vi "KB-CalConcentrieity.vi"(0 "Image  In":T5(plugin-control), 1 "ROI Descriptor (Otter-Find Circular Edge)":T1={"Global Rectangle"=[686, 409, 1084, 806], "Contours"=[{"ID"=enum."External", "Type"=7, "Coordinates"=[884, 607, 109, 198, 0, 0]}]} {"Contours"."Type" items=["No Selection", "Point", "Line", "Rectangle", "Oval", "Polygon", "Freehand Region", "Annulus", "Unused2", "Unused3", "Broken Line", "Freehand Line", "Rotated Rectangle"]}, 2 "Options (Otter-Find Circular Edge)":T4={"Search  Direction"=0, "Edge Options"={"Edge Polarity"=0, "Kernel Size"=13, "Width"=13, "Minimum Edge Strength"=53.0, "Interpolation Type"=enum."Bilinear Fixed", "Data Processing Method"=enum."Average"}, "Show Search Area"=TRUE, "Show Search Lines"=TRUE, "Show Edges Found"=TRUE, "Show Result"=TRUE, "Search Area Color"=65280, "Search Lines Color"=255, "Edge Locations Color"=16776960, "Result Color"=16711680, "Overlay Group Name"=""} {"Search  Direction" items=["Outside to Inside", "Inside to Outside"]; "Edge Options"."Edge Polarity" items=["All Edges", "Rising Edges", "Falling Edges"]; "Edge Options"."Minimum Edge Strength" format="%.2f"; "Edge Options"."Width" step=2; "Edge Options"."Kernel Size" step=2}, 3 "ROI Descriptor (Inner Find Circular Edge 2)":T1={"Global Rectangle"=[775, 498, 995, 717], "Contours"=[{"ID"=enum."External", "Type"=7, "Coordinates"=[884, 607, 51, 109, 0, 0]}]} {"Contours"."Type" items=["No Selection", "Point", "Line", "Rectangle", "Oval", "Polygon", "Freehand Region", "Annulus", "Unused2", "Unused3", "Broken Line", "Freehand Line", "Rotated Rectangle"]}, 4 "Options (Inner Find Circular Edge 2)":T4={"Search  Direction"=0, "Edge Options"={"Edge Polarity"=0, "Kernel Size"=13, "Width"=13, "Minimum Edge Strength"=72.0, "Interpolation Type"=enum."Bilinear Fixed", "Data Processing Method"=enum."Average"}, "Show Search Area"=TRUE, "Show Search Lines"=TRUE, "Show Edges Found"=TRUE, "Show Result"=TRUE, "Search Area Color"=65280, "Search Lines Color"=255, "Edge Locations Color"=16776960, "Result Color"=16711680, "Overlay Group Name"=""} {"Search  Direction" items=["Outside to Inside", "Inside to Outside"]; "Edge Options"."Edge Polarity" items=["All Edges", "Rising Edges", "Falling Edges"]; "Edge Options"."Minimum Edge Strength" format="%.2f"; "Edge Options"."Width" step=2; "Edge Options"."Kernel Size" step=2}, 5 "error in":errorcluster, 6 "Row Select":string(combo)="Item1", 7 "Range (Threshold 1)":cluster{"Lower value":sgl, "Upper value":sgl}={"Lower value"=218.0, "Upper value"=255.0}, 8 "相机分辨率":string) -> (13 "U I Center":cluster{"X":sgl, "Y":sgl}[](array[cluster]), 14 "Image  Out":T5(plugin-control), 16 "Concentrieity":string, 17 "color":string, 18 "New Inneer ROI":T1, 19 "error out":errorcluster)   [LabVIEW 2015]
uses:
  <vilib>/vision/Measure.llb/Edge Options.ctl
  <vilib>/vision/Measure.llb/Edge Polarity.ctl
  Global System.vi
panel:
  out "New Inneer ROI 2":T1
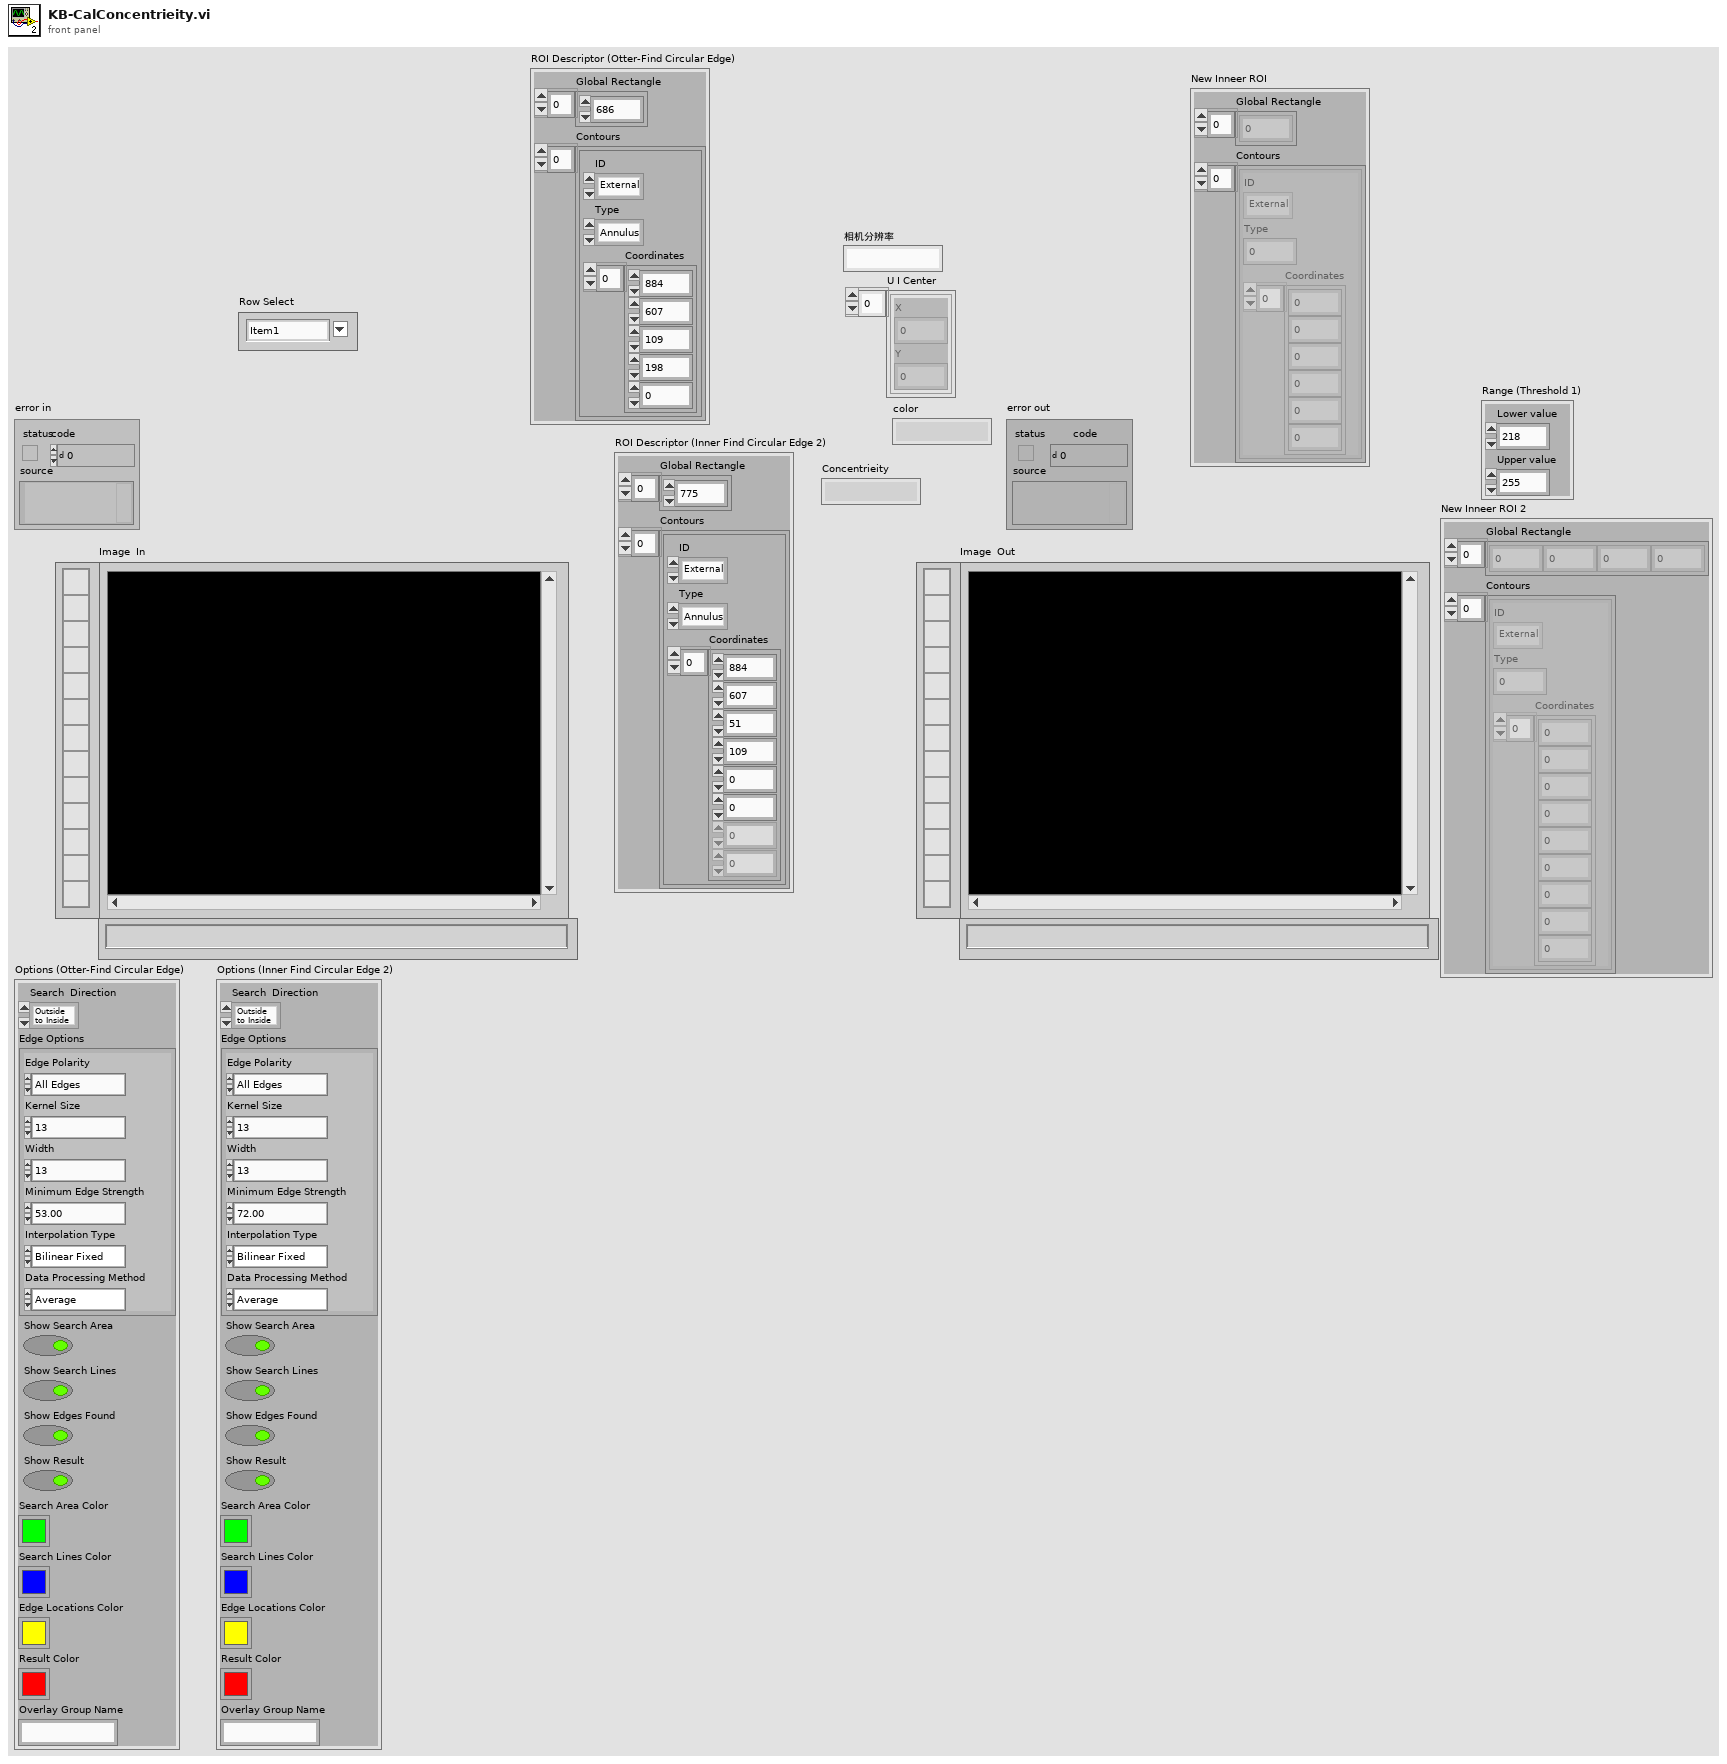
[diagram p1: front panel]
types:
  T1 = cluster{"Global Rectangle":i32[], "Contours":cluster{"ID":enum32{"External", "Internal"}, "Type":u32, "Coordinates":i32[]}[]}
  T2 = typedef "Edge Options.ctl" = cluster{"Edge Polarity":T3, "Kernel Size":u32, "Width":u32, "Minimum Edge Strength":sgl, "Interpolation Type":enum32{"Zero Order", "Bilinear", "Quadratic", "Cubic", "Bilinear Fixed"}, "Data Processing Method":enum32{"Average", "Median"}}
  T3 = typedef "Edge Polarity.ctl" = u32
  T4 = cluster{"Search  Direction":u32, "Edge Options":T2, "Show Search Area":bool, "Show Search Lines":bool, "Show Edges Found":bool, "Show Result":bool, "Search Area Color":u32, "Search Lines Color":u32, "Edge Locations Color":u32, "Result Color":u32, "Overlay Group Name":string}
  T5 = typedef "IMAQ Image.ctl" = refnum<image>
  T6 = cluster{"Left":i32, "Top":i32, "Right":i32, "Bottom":i32}
  T7 = typedef "Image Type" = u32
  T8 = cluster{"ID":enum32{"External", "Internal"}, "Type":u32, "Coordinates":i32[]}
  T9 = cluster{"Process":enum16{"Get First Edge", "Get First + Last Edge", "Get All Edges", "Get Best Edge"}, "Step Size":i32, "Max Pixel Radius":i32}
  T10 = cluster{"Center (Pixels)":cluster{"X":sgl, "Y":sgl}, "Radius (Pixels)":dbl, "Center (Real-World)":cluster{"X":sgl, "Y":sgl}, "Radius (Real-World)":dbl, "Roundness (Real-World)":dbl, "Average Strength":dbl, "Average SNR (dB)":dbl}
  T11 = cluster{"left":dbl, "top":dbl, "right":dbl, "bottom":dbl}
  T12 = cluster{"ID":enum32{"External", "Internal"}, "Type":u32, "Coordinates":i32[]}[]
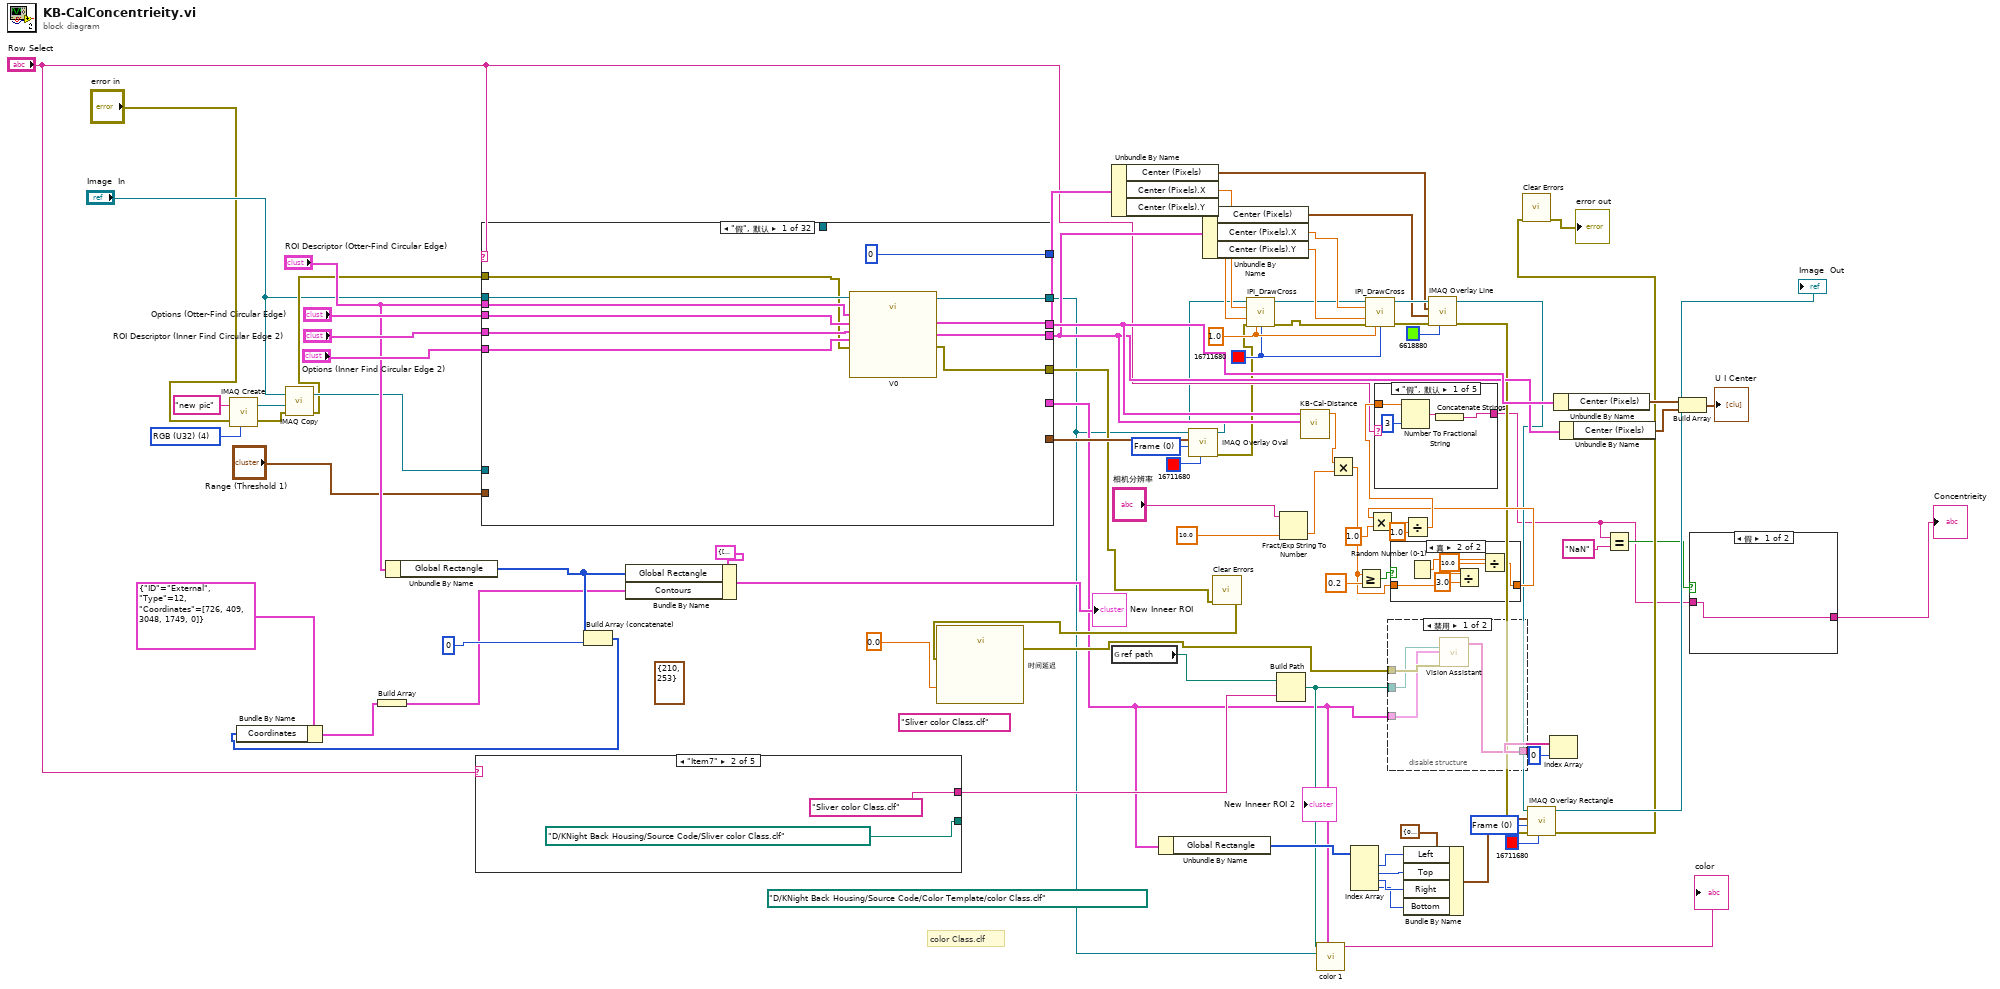
[diagram p0: block diagram]
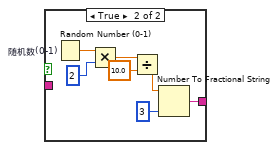
[diagram p2: hidden frame]
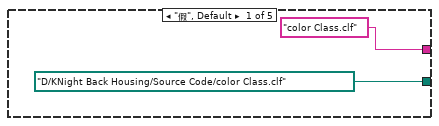
[diagram p4: hidden frame]
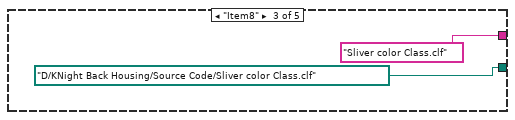
[diagram p5: hidden frame]
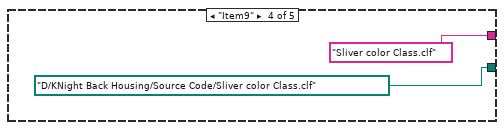
[diagram p6: hidden frame]
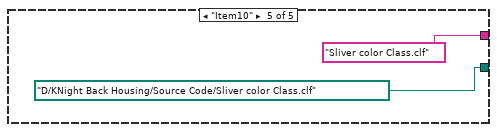
[diagram p7: hidden frame]
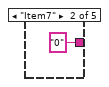
[diagram p9: hidden frame]
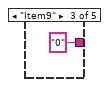
[diagram p10: hidden frame]
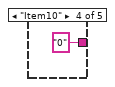
[diagram p11: hidden frame]
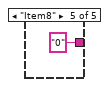
[diagram p12: hidden frame]
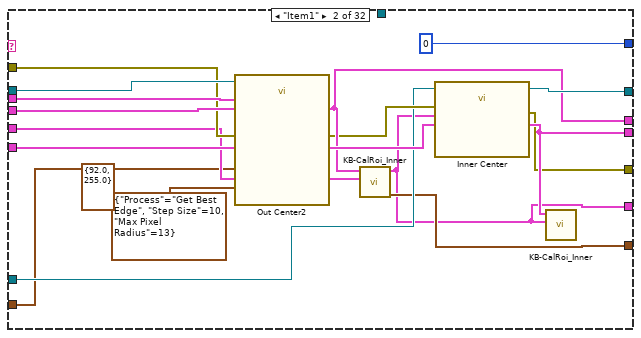
[diagram p13: hidden frame]
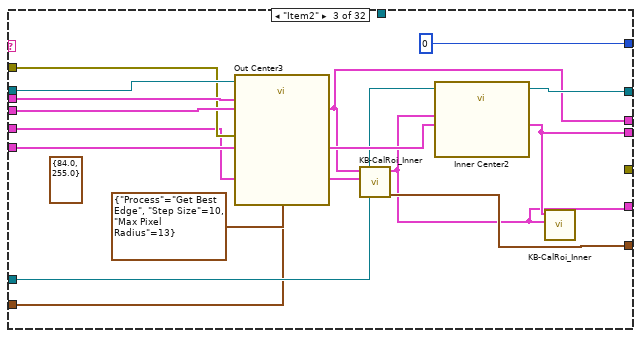
[diagram p14: hidden frame]
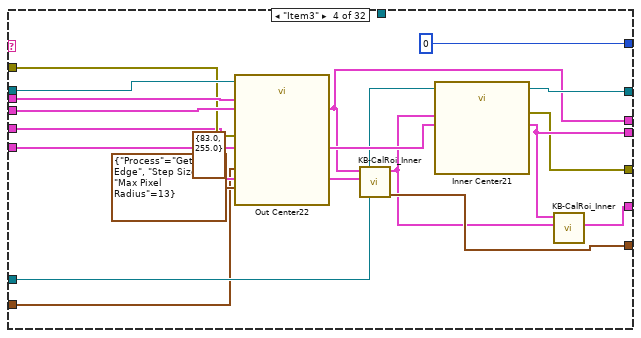
[diagram p15: hidden frame]
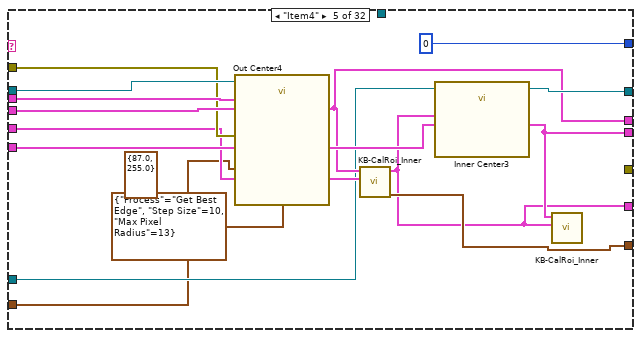
[diagram p16: hidden frame]
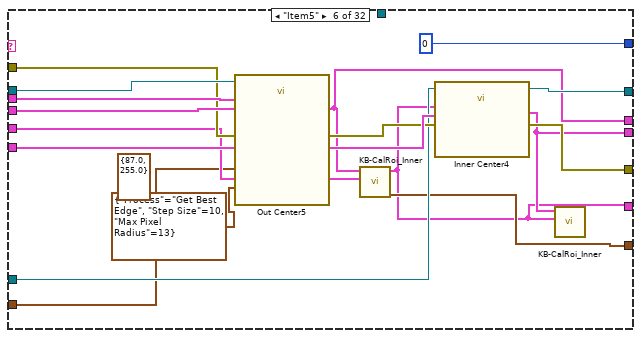
[diagram p17: hidden frame]
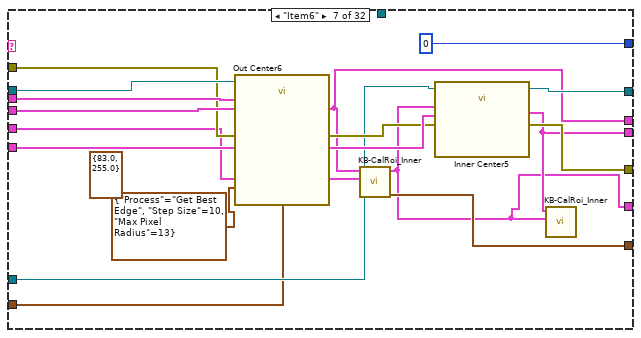
[diagram p18: hidden frame]
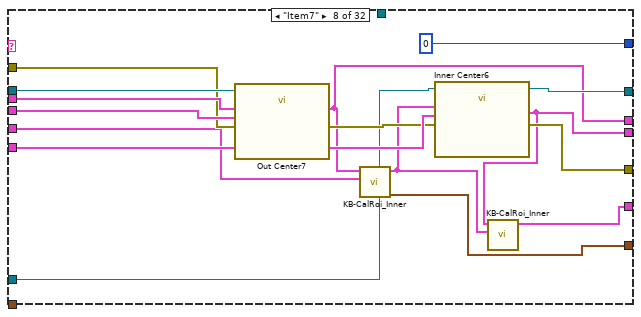
[diagram p19: hidden frame]
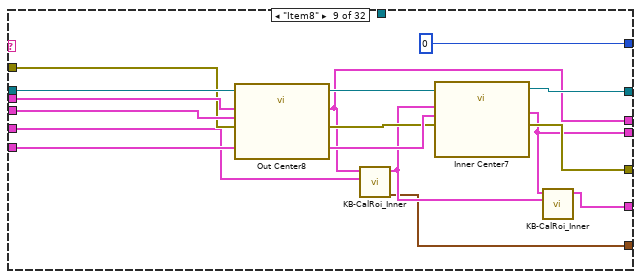
[diagram p20: hidden frame]
diagram:
  (unwired) "Sliver color Class.clf" ("名称或相对路径")
  w24 = u32 0 items=["Frame", "Fill", "Highlight"] ("Drawing Mode (Frame)")
  w40 = u32 0 items=["Frame", "Fill"] ("Drawing Mode (Frame)")
  (unwired) path "D:/KNight Back Housing/Source Code/Color Template/color Class.clf" ("File Path (Color Classification 1)")
  (unwired) cluster{"Lower value":i32, "Upper value":i32} {"Lower value"=210, "Upper value"=253} ("Red or Hue Range (Color Threshold 1) 3")
  w47 = T7 4 items=["Grayscale (U8)", "Grayscale (I16)", "Grayscale (SGL)", "Complex (CSG)", "RGB (U32)", "HSL (U32)", "RGB (U64)", "Grayscale (U16)"] ("Image Type")
  w69 = u32 16711680 ("颜色盒")
  w70 = 1.0 ("Radius")
  # "color Class.clf"
  n1 = call "IMAQ Create"("Image Name"="new pic", "Image Type"=w47, "error in (no error)"="error in") -> ("New Image"=w46:T5, "error out"=w45:errorcluster)  [unwired: 2 in]
  n2 = call "IMAQ Copy"("error in (no error)"=w45, "Image Dst"=w46, "Image Src"="Image  In") -> ("error out"=w16:errorcluster, "Image Dst Out"=w17:T5)  [unwired: 3 in]
  n3 = Unbundle By Name("ROI Descriptor (Otter-Find Circular Edge)") -> ("Global Rectangle"=w59:i32[])
  n4 = case shown="\"Item7\"" "Row Select" {
    tunnel: ["color Class.clf" ("名称或相对路径") "Sliver color Class.clf" ("名称或相对路径") "Sliver color Class.clf" ("名称或相对路径") "Sliver color Class.clf" ("名称或相对路径") "Sliver color Class.clf" ("名称或相对路径")] -> w19
    tunnel: [path "D:/KNight Back Housing/Source Code/color Class.clf" ("File Path (Color Classification 1)") path "D:/KNight Back Housing/Source Code/Sliver color Class.clf" ("File Path (Color Classification 1)") path "D:/KNight Back Housing/Source Code/Sliver color Class.clf" ("File Path (Color Classification 1)") path "D:/KNight Back Housing/Source Code/Sliver color Class.clf" ("File Path (Color Classification 1)") path "D:/KNight Back Housing/Source Code/Sliver color Class.clf" ("File Path (Color Classification 1)")] -> _
    frame "假", Default {
    }
    frame "Item7" {
    }
    frame "Item8" {
    }
    frame "Item9" {
    }
    frame "Item10" {
    }
  }
  n5 = case shown="\"假\", 默认" "Row Select" {
    tunnel: [0 0 0 0 0 0 0 0 0 0 0 0 0 0 0 0 0 0 0 0 0 0 0 0 0 0 0 0 0 0 0 0] -> _
    tunnel: "Image  In" -> [w107 w122 w137 w153 w168 w184 w201 w217 w233 w249 w265 w281 w296 w311 w326 w341 w357 w372 w388 w404 w420 w436 w455 w463 w491 w509 w527 w544 w561 w578 w595 w613]
    tunnel: "ROI Descriptor (Otter-Find Circular Edge)" -> [w106 w121 w136 w152 w167 w183 w200 w216 w231 w247 w263 w280 w295 w310 w325 w340 w356 w371 w387 w403 w419 w435 w454 w473 w490 w508 w526 w543 w560 w577 w594 w612]
    tunnel: "Options (Otter-Find Circular Edge)" -> [w105 w120 w135 w151 w166 w182 w199 w215 w230 w246 w262 w279 w294 w309 w324 w339 w355 w370 w386 w402 w418 w434 w453 w472 w489 w507 w525 w542 w559 w576 w593 w611]
    tunnel: "ROI Descriptor (Inner Find Circular Edge 2)" -> [w104 w118 w133 w149 w164 w179 w196 w212 w227 w243 w259 w277 w292 w307 w322 w337 w353 w368 w384 w400 w416 w432 w451 w470 w487 w505 w515 w540 w557 w574 w591 w609]
    tunnel: "Options (Inner Find Circular Edge 2)" -> [w103 w124 w139 w155 w170 w187 w204 w220 w236 w252 w268 w283 w298 w313 w328 w343 w359 w374 w390 w406 w422 w438 w456 w474 w492 w510 w528 w545 w562 w579 w596 w614]
    tunnel: [w101 w123 w138 w154 w169 w186 w203 w219 w235 w251 w267 w282 w297 w312 w327 w342 w358 w373 w389 w405 w421 w437 w441 w459 w477 w495 w513 w530 w547 w565 w583 w598] -> w5
    tunnel: [w100 w117 w132 w148 w163 w178 w195 w211 w226 w242 w258 w276 w291 w306 w321 w336 w352 w367 w383 w399 w415 w431 w450 w469 w486 w504 w522 w539 w556 w573 w590 w608] -> w76
    tunnel: [w99 w116 w131 w147 w162 w177 w194 w210 w225 w241 w257 w275 w290 w305 w320 w335 w351 w366 w382 w398 w414 w430 w449 w462 w485 w503 w520 w538 w555 w572 w589 w607] -> w73
    tunnel: w16 -> [w102 w119 w134 w150 w165 w181 w198 w214 w229 w245 w261 w278 w293 w308 w323 w338 w354 w369 w385 w401 w417 w433 w452 w471 w488 w506 w524 w541 w558 w575 w592 w610]
    tunnel: [w98 w114 _ w145 _ w185 w202 w218 w234 w250 w266 _ _ _ _ _ _ _ _ _ _ _ w440 w460 w476 w496 w512 w531 w548 w564 w582 w599] -> w14
    tunnel: [_ w109 w126 w141 w157 w172 w189 w206 w223 w239 w255 w270 w285 w300 w315 w330 w345 w361 w376 w392 w408 w424 w443 w461 w479 w497 w515 w533 w550 w567 w584 w601] -> w7
    tunnel: w17 -> [_ w112 w130 w144 w160 w176 w193 w207 _ _ _ w273 w289 w303 w318 w334 w350 w364 w380 w397 w413 w429 w448 w465 w484 w501 w518 w537 w554 w570 w587 w603]
    tunnel: "Range (Threshold 1)" -> [_ w111 w127 w142 w158 w173 w190 _ _ _ _ w271 w286 w301 w316 w331 w347 w362 w378 w394 w410 w426 w444 w464 w480 w498 w516 w534 w551 w568 w585 w602]
    tunnel: [_ w110 w129 w146 w161 w175 w192 w208 w222 w238 w254 w274 w288 w304 w319 w333 w349 w365 w381 w396 w412 w428 w442 w458 w478 w494 w514 w532 w549 w566 w581 w600] -> w38
    tunnel: [_ _ _ _ _ _ _ _ _ _ _ _ _ _ _ _ w346 _ w377 w393 w409 w425 _ _ _ _ _ _ _ _ _ _] -> _
    frame "假", Default {
      n6 = call "V0"("Image In"=w107, "ROI Descriptor (Otter-Find Circular Edge)"=w106, "Options (Otter-Find Circular Edge)"=w105, "ROI Descriptor (Inner Find Circular Edge 2)"=w104, "Options (Inner Find Circular Edge 2)"=w103, "error in"=w102) -> ("Image Out"=w101:T5, "Fitted Circle (Otter-Find Circular Edge)"=w100:T10, "Fitted Circle (Inner Find Circular Edge 2)"=w99:T10, "error out"=w98:errorcluster)  [unwired: 17 in, 1 out]
    }
    frame "Item1" {
      (unwired) cluster{"Lower value":sgl, "Upper value":sgl} {"Lower value"=92.0, "Upper value"=255.0} ("Range (Threshold 1)")
      n7 = call "Out Center2"("Image In"=w122, "ROI Descriptor (Otter-Find Circular Edge)"=w121, "Options (Otter-Find Circular Edge)"=w120, "Range (Threshold 1)"=w111, "Circle Fit Options (Otter-Find Circular Edge)"=T9 {"Process"=enum."Get Best Edge", "Step Size"=10, "Max Pixel Radius"=13}, "error in"=w119) -> ("Fitted Circle (Otter-Find Circular Edge)"=w117:T10, "error out"=w115:errorcluster)  [unwired: 19 in, 1 out]
      n8 = call "KB-CalRoi_Inner.vi"("Inner ROI Descriptor (Inner Find Circular Edge 2)"=w118, "Fitted Circle (Otter-Find Circular Edge)"=w117) -> ("Roi"=w110:T11, "New Inneer ROI"=w109:T1)  [unwired: 8 in]
      n9 = call "Inner Center"("Image In"=w112, "error in"=w115, "ROI Descriptor (Inner Find Circular Edge 2)"=w109, "Options (Inner Find Circular Edge 2)"=w124) -> ("Image Out"=w123:T5, "error out"=w114:errorcluster, "Fitted Circle (Inner Find Circular Edge 2)"=w116:T10)  [unwired: 20 in, 1 out]
      n10 = call "KB-CalRoi_Inner.vi"("Inner ROI Descriptor (Inner Find Circular Edge 2)"=w109, "Fitted Circle (Otter-Find Circular Edge)"=w116) -> ()  [unwired: 8 in, 2 out]
    }
    frame "Item2" {
      (unwired) cluster{"Lower value":sgl, "Upper value":sgl} {"Lower value"=84.0, "Upper value"=255.0} ("Range (Threshold 1)")
      n11 = call "Out Center3"("Image In"=w137, "ROI Descriptor (Otter-Find Circular Edge)"=w136, "Options (Otter-Find Circular Edge)"=w135, "Range (Threshold 1)"=w127, "Circle Fit Options (Otter-Find Circular Edge)"=T9 {"Process"=enum."Get Best Edge", "Step Size"=10, "Max Pixel Radius"=13}, "error in"=w134) -> ("Fitted Circle (Otter-Find Circular Edge)"=w132:T10)  [unwired: 19 in, 2 out]
      n12 = call "KB-CalRoi_Inner.vi"("Inner ROI Descriptor (Inner Find Circular Edge 2)"=w133, "Fitted Circle (Otter-Find Circular Edge)"=w132) -> ("Roi"=w129:T11, "New Inneer ROI"=w126:T1)  [unwired: 8 in]
      n13 = call "Inner Center2"("Image In"=w130, "ROI Descriptor (Inner Find Circular Edge 2)"=w126, "Options (Inner Find Circular Edge 2)"=w139) -> ("Image Out"=w138:T5, "Fitted Circle (Inner Find Circular Edge 2)"=w131:T10)  [unwired: 21 in, 2 out]
      n14 = call "KB-CalRoi_Inner.vi"("Inner ROI Descriptor (Inner Find Circular Edge 2)"=w126, "Fitted Circle (Otter-Find Circular Edge)"=w131) -> ()  [unwired: 8 in, 2 out]
    }
    frame "Item3" {
      (unwired) cluster{"Lower value":sgl, "Upper value":sgl} {"Lower value"=83.0, "Upper value"=255.0} ("Range (Threshold 1)")
      n15 = call "Out Center22"("Image In"=w153, "ROI Descriptor (Otter-Find Circular Edge)"=w152, "Options (Otter-Find Circular Edge)"=w151, "Range (Threshold 1)"=w142, "Circle Fit Options (Otter-Find Circular Edge)"=T9 {"Process"=enum."Get Best Edge", "Step Size"=10, "Max Pixel Radius"=13}, "error in"=w150) -> ("Fitted Circle (Otter-Find Circular Edge)"=w148:T10)  [unwired: 19 in, 2 out]
      n16 = call "KB-CalRoi_Inner.vi"("Inner ROI Descriptor (Inner Find Circular Edge 2)"=w149, "Fitted Circle (Otter-Find Circular Edge)"=w148) -> ("Roi"=w146:T11, "New Inneer ROI"=w141:T1)  [unwired: 8 in]
      n17 = call "Inner Center21"("Image In"=w144, "ROI Descriptor (Inner Find Circular Edge 2)"=w141, "Options (Inner Find Circular Edge 2)"=w155) -> ("Image Out"=w154:T5, "error out"=w145:errorcluster, "Fitted Circle (Inner Find Circular Edge 2)"=w147:T10)  [unwired: 21 in, 1 out]
      n18 = call "KB-CalRoi_Inner.vi"("Inner ROI Descriptor (Inner Find Circular Edge 2)"=w141, "Fitted Circle (Otter-Find Circular Edge)"=w147) -> ()  [unwired: 8 in, 2 out]
    }
    frame "Item4" {
      (unwired) cluster{"Lower value":sgl, "Upper value":sgl} {"Lower value"=87.0, "Upper value"=255.0} ("Range (Threshold 1)")
      n19 = call "Out Center4"("Image In"=w168, "ROI Descriptor (Otter-Find Circular Edge)"=w167, "Options (Otter-Find Circular Edge)"=w166, "Range (Threshold 1)"=w158, "Circle Fit Options (Otter-Find Circular Edge)"=T9 {"Process"=enum."Get Best Edge", "Step Size"=10, "Max Pixel Radius"=13}, "error in"=w165) -> ("Fitted Circle (Otter-Find Circular Edge)"=w163:T10)  [unwired: 19 in, 2 out]
      n20 = call "KB-CalRoi_Inner.vi"("Inner ROI Descriptor (Inner Find Circular Edge 2)"=w164, "Fitted Circle (Otter-Find Circular Edge)"=w163) -> ("Roi"=w161:T11, "New Inneer ROI"=w157:T1)  [unwired: 8 in]
      n21 = call "Inner Center3"("Image In"=w160, "ROI Descriptor (Inner Find Circular Edge 2)"=w157, "Options (Inner Find Circular Edge 2)"=w170) -> ("Image Out"=w169:T5, "Fitted Circle (Inner Find Circular Edge 2)"=w162:T10)  [unwired: 21 in, 2 out]
      n22 = call "KB-CalRoi_Inner.vi"("Inner ROI Descriptor (Inner Find Circular Edge 2)"=w157, "Fitted Circle (Otter-Find Circular Edge)"=w162) -> ()  [unwired: 8 in, 2 out]
    }
    frame "Item5" {
      (unwired) cluster{"Lower value":sgl, "Upper value":sgl} {"Lower value"=87.0, "Upper value"=255.0} ("Range (Threshold 1)")
      n23 = call "Out Center5"("Image In"=w184, "ROI Descriptor (Otter-Find Circular Edge)"=w183, "Options (Otter-Find Circular Edge)"=w182, "Range (Threshold 1)"=w173, "Circle Fit Options (Otter-Find Circular Edge)"=T9 {"Process"=enum."Get Best Edge", "Step Size"=10, "Max Pixel Radius"=13}, "error in"=w181) -> ("Fitted Circle (Otter-Find Circular Edge)"=w178:T10, "error out"=w180:errorcluster)  [unwired: 19 in, 1 out]
      n24 = call "KB-CalRoi_Inner.vi"("Inner ROI Descriptor (Inner Find Circular Edge 2)"=w179, "Fitted Circle (Otter-Find Circular Edge)"=w178) -> ("Roi"=w175:T11, "New Inneer ROI"=w172:T1)  [unwired: 8 in]
      n25 = call "Inner Center4"("Image In"=w176, "ROI Descriptor (Inner Find Circular Edge 2)"=w172, "Options (Inner Find Circular Edge 2)"=w187, "error in"=w180) -> ("Image Out"=w186:T5, "Fitted Circle (Inner Find Circular Edge 2)"=w177:T10, "error out"=w185:errorcluster)  [unwired: 20 in, 1 out]
      n26 = call "KB-CalRoi_Inner.vi"("Inner ROI Descriptor (Inner Find Circular Edge 2)"=w172, "Fitted Circle (Otter-Find Circular Edge)"=w177) -> ()  [unwired: 8 in, 2 out]
    }
    frame "Item6" {
      (unwired) cluster{"Lower value":sgl, "Upper value":sgl} {"Lower value"=83.0, "Upper value"=255.0} ("Range (Threshold 1)")
      n27 = call "Out Center6"("Image In"=w201, "ROI Descriptor (Otter-Find Circular Edge)"=w200, "Options (Otter-Find Circular Edge)"=w199, "Range (Threshold 1)"=w190, "Circle Fit Options (Otter-Find Circular Edge)"=T9 {"Process"=enum."Get Best Edge", "Step Size"=10, "Max Pixel Radius"=13}, "error in"=w198) -> ("Fitted Circle (Otter-Find Circular Edge)"=w195:T10, "error out"=w197:errorcluster)  [unwired: 19 in, 1 out]
      n28 = call "KB-CalRoi_Inner.vi"("Inner ROI Descriptor (Inner Find Circular Edge 2)"=w196, "Fitted Circle (Otter-Find Circular Edge)"=w195) -> ("Roi"=w192:T11, "New Inneer ROI"=w189:T1)  [unwired: 8 in]
      n29 = call "Inner Center5"("Image In"=w193, "ROI Descriptor (Inner Find Circular Edge 2)"=w189, "Options (Inner Find Circular Edge 2)"=w204, "error in"=w197) -> ("Image Out"=w203:T5, "Fitted Circle (Inner Find Circular Edge 2)"=w194:T10, "error out"=w202:errorcluster)  [unwired: 20 in, 1 out]
      n30 = call "KB-CalRoi_Inner.vi"("Inner ROI Descriptor (Inner Find Circular Edge 2)"=w189, "Fitted Circle (Otter-Find Circular Edge)"=w194) -> ()  [unwired: 8 in, 2 out]
    }
    frame "Item7" {
      n31 = call "Out Center7"("Image In"=w217, "ROI Descriptor (Otter-Find Circular Edge)"=w216, "Options (Otter-Find Circular Edge)"=w215, "error in"=w214) -> ("Fitted Circle (Otter-Find Circular Edge)"=w211:T10, "error out"=w213:errorcluster)  [unwired: 21 in, 1 out]
      n32 = call "KB-CalRoi_Inner.vi"("Inner ROI Descriptor (Inner Find Circular Edge 2)"=w212, "Fitted Circle (Otter-Find Circular Edge)"=w211) -> ("Roi"=w208:T11, "New Inneer ROI"=w209:T1)  [unwired: 8 in]
      n33 = call "Inner Center6"("Image In"=w207, "ROI Descriptor (Inner Find Circular Edge 2)"=w209, "Options (Inner Find Circular Edge 2)"=w220, "error in"=w213) -> ("Image Out"=w219:T5, "Fitted Circle (Inner Find Circular Edge 2)"=w210:T10, "error out"=w218:errorcluster)  [unwired: 20 in, 1 out]
      n34 = call "KB-CalRoi_Inner.vi"("Inner ROI Descriptor (Inner Find Circular Edge 2)"=w209, "Fitted Circle (Otter-Find Circular Edge)"=w210) -> ("New Inneer ROI"=w206:T1)  [unwired: 8 in, 1 out]
    }
    frame "Item8" {
      n35 = call "Out Center8"("Image In"=w233, "ROI Descriptor (Otter-Find Circular Edge)"=w231, "Options (Otter-Find Circular Edge)"=w230, "error in"=w229) -> ("Image Out"=w232:T5, "Fitted Circle (Otter-Find Circular Edge)"=w226:T10, "error out"=w228:errorcluster)  [unwired: 21 in]
      n36 = call "KB-CalRoi_Inner.vi"("Inner ROI Descriptor (Inner Find Circular Edge 2)"=w227, "Fitted Circle (Otter-Find Circular Edge)"=w226) -> ("Roi"=w222:T11, "New Inneer ROI"=w224:T1)  [unwired: 8 in]
      n37 = call "Inner Center7"("Image In"=w232, "ROI Descriptor (Inner Find Circular Edge 2)"=w224, "Options (Inner Find Circular Edge 2)"=w236, "error in"=w228) -> ("Image Out"=w235:T5, "Fitted Circle (Inner Find Circular Edge 2)"=w225:T10, "error out"=w234:errorcluster)  [unwired: 20 in, 1 out]
      n38 = call "KB-CalRoi_Inner.vi"("Inner ROI Descriptor (Inner Find Circular Edge 2)"=w224, "Fitted Circle (Otter-Find Circular Edge)"=w225) -> ("New Inneer ROI"=w223:T1)  [unwired: 8 in, 1 out]
    }
    frame "Item9" {
      n39 = call "Out Center9"("Image In"=w249, "ROI Descriptor (Otter-Find Circular Edge)"=w247, "Options (Otter-Find Circular Edge)"=w246, "error in"=w245) -> ("Image Out"=w248:T5, "Fitted Circle (Otter-Find Circular Edge)"=w242:T10, "error out"=w244:errorcluster)  [unwired: 21 in]
      n40 = call "KB-CalRoi_Inner.vi"("Inner ROI Descriptor (Inner Find Circular Edge 2)"=w243, "Fitted Circle (Otter-Find Circular Edge)"=w242) -> ("Roi"=w238:T11, "New Inneer ROI"=w240:T1)  [unwired: 8 in]
      n41 = call "Inner Center8"("Image In"=w248, "ROI Descriptor (Inner Find Circular Edge 2)"=w240, "Options (Inner Find Circular Edge 2)"=w252, "error in"=w244) -> ("Image Out"=w251:T5, "Fitted Circle (Inner Find Circular Edge 2)"=w241:T10, "error out"=w250:errorcluster)  [unwired: 20 in, 1 out]
      n42 = call "KB-CalRoi_Inner.vi"("Inner ROI Descriptor (Inner Find Circular Edge 2)"=w240, "Fitted Circle (Otter-Find Circular Edge)"=w241) -> ("New Inneer ROI"=w239:T1)  [unwired: 8 in, 1 out]
    }
    frame "Item10" {
      n43 = call "Out Center10"("Image In"=w265, "ROI Descriptor (Otter-Find Circular Edge)"=w263, "Options (Otter-Find Circular Edge)"=w262, "error in"=w261) -> ("Image Out"=w264:T5, "Fitted Circle (Otter-Find Circular Edge)"=w258:T10, "error out"=w260:errorcluster)  [unwired: 21 in]
      n44 = call "KB-CalRoi_Inner.vi"("Inner ROI Descriptor (Inner Find Circular Edge 2)"=w259, "Fitted Circle (Otter-Find Circular Edge)"=w258) -> ("Roi"=w254:T11, "New Inneer ROI"=w256:T1)  [unwired: 8 in]
      n45 = call "Inner Center9"("Image In"=w264, "ROI Descriptor (Inner Find Circular Edge 2)"=w256, "Options (Inner Find Circular Edge 2)"=w268, "error in"=w260) -> ("Image Out"=w267:T5, "Fitted Circle (Inner Find Circular Edge 2)"=w257:T10, "error out"=w266:errorcluster)  [unwired: 20 in, 1 out]
      n46 = call "KB-CalRoi_Inner.vi"("Inner ROI Descriptor (Inner Find Circular Edge 2)"=w256, "Fitted Circle (Otter-Find Circular Edge)"=w257) -> ("New Inneer ROI"=w255:T1)  [unwired: 8 in, 1 out]
    }
    frame "Item11" {
      (unwired) cluster{"Lower value":sgl, "Upper value":sgl} {"Lower value"=92.0, "Upper value"=255.0} ("Range (Threshold 1)")
      n47 = call "Out Center11"("Image In"=w281, "ROI Descriptor (Otter-Find Circular Edge)"=w280, "Options (Otter-Find Circular Edge)"=w279, "Range (Threshold 1)"=w271, "Circle Fit Options (Otter-Find Circular Edge)"=T9 {"Process"=enum."Get Best Edge", "Step Size"=10, "Max Pixel Radius"=13}, "error in"=w278) -> ("Fitted Circle (Otter-Find Circular Edge)"=w276:T10)  [unwired: 19 in, 2 out]
      n48 = call "KB-CalRoi_Inner.vi"("Inner ROI Descriptor (Inner Find Circular Edge 2)"=w277, "Fitted Circle (Otter-Find Circular Edge)"=w276) -> ("Roi"=w274:T11, "New Inneer ROI"=w270:T1)  [unwired: 8 in]
      n49 = call "Inner Center10"("Image In"=w273, "ROI Descriptor (Inner Find Circular Edge 2)"=w270, "Options (Inner Find Circular Edge 2)"=w283) -> ("Image Out"=w282:T5, "Fitted Circle (Inner Find Circular Edge 2)"=w275:T10)  [unwired: 21 in, 2 out]
      n50 = call "KB-CalRoi_Inner.vi"("Inner ROI Descriptor (Inner Find Circular Edge 2)"=w270, "Fitted Circle (Otter-Find Circular Edge)"=w275) -> ()  [unwired: 8 in, 2 out]
    }
    frame "Item12" {
      (unwired) cluster{"Lower value":sgl, "Upper value":sgl} {"Lower value"=94.0, "Upper value"=255.0} ("Range (Threshold 1)")
      n51 = call "Out Center12"("Image In"=w296, "ROI Descriptor (Otter-Find Circular Edge)"=w295, "Options (Otter-Find Circular Edge)"=w294, "Range (Threshold 1)"=w286, "Circle Fit Options (Otter-Find Circular Edge)"=T9 {"Process"=enum."Get Best Edge", "Step Size"=10, "Max Pixel Radius"=13}, "error in"=w293) -> ("Fitted Circle (Otter-Find Circular Edge)"=w291:T10)  [unwired: 19 in, 2 out]
      n52 = call "KB-CalRoi_Inner.vi"("Inner ROI Descriptor (Inner Find Circular Edge 2)"=w292, "Fitted Circle (Otter-Find Circular Edge)"=w291) -> ("Roi"=w288:T11, "New Inneer ROI"=w285:T1)  [unwired: 8 in]
      n53 = call "Inner Center11"("Image In"=w289, "ROI Descriptor (Inner Find Circular Edge 2)"=w285, "Options (Inner Find Circular Edge 2)"=w298) -> ("Image Out"=w297:T5, "Fitted Circle (Inner Find Circular Edge 2)"=w290:T10)  [unwired: 21 in, 2 out]
      n54 = call "KB-CalRoi_Inner.vi"("Inner ROI Descriptor (Inner Find Circular Edge 2)"=w285, "Fitted Circle (Otter-Find Circular Edge)"=w290) -> ()  [unwired: 8 in, 2 out]
    }
    frame "Item13" {
      (unwired) cluster{"Lower value":sgl, "Upper value":sgl} {"Lower value"=92.0, "Upper value"=255.0} ("Range (Threshold 1)")
      n55 = call "Out Center13"("Image In"=w311, "ROI Descriptor (Otter-Find Circular Edge)"=w310, "Options (Otter-Find Circular Edge)"=w309, "Range (Threshold 1)"=w301, "Circle Fit Options (Otter-Find Circular Edge)"=T9 {"Process"=enum."Get Best Edge", "Step Size"=10, "Max Pixel Radius"=13}, "error in"=w308) -> ("Fitted Circle (Otter-Find Circular Edge)"=w306:T10)  [unwired: 19 in, 2 out]
      n56 = call "KB-CalRoi_Inner.vi"("Inner ROI Descriptor (Inner Find Circular Edge 2)"=w307, "Fitted Circle (Otter-Find Circular Edge)"=w306) -> ("Roi"=w304:T11, "New Inneer ROI"=w300:T1)  [unwired: 8 in]
      n57 = call "Inner Center12"("Image In"=w303, "ROI Descriptor (Inner Find Circular Edge 2)"=w300, "Options (Inner Find Circular Edge 2)"=w313) -> ("Image Out"=w312:T5, "Fitted Circle (Inner Find Circular Edge 2)"=w305:T10)  [unwired: 21 in, 2 out]
      n58 = call "KB-CalRoi_Inner.vi"("Inner ROI Descriptor (Inner Find Circular Edge 2)"=w300, "Fitted Circle (Otter-Find Circular Edge)"=w305) -> ()  [unwired: 8 in, 2 out]
    }
    frame "Item14" {
      (unwired) cluster{"Lower value":sgl, "Upper value":sgl} {"Lower value"=96.0, "Upper value"=255.0} ("Range (Threshold 1)")
      n59 = call "Out Center14"("Image In"=w326, "ROI Descriptor (Otter-Find Circular Edge)"=w325, "Options (Otter-Find Circular Edge)"=w324, "Range (Threshold 1)"=w316, "Circle Fit Options (Otter-Find Circular Edge)"=T9 {"Process"=enum."Get Best Edge", "Step Size"=10, "Max Pixel Radius"=13}, "error in"=w323) -> ("Fitted Circle (Otter-Find Circular Edge)"=w321:T10)  [unwired: 19 in, 2 out]
      n60 = call "KB-CalRoi_Inner.vi"("Inner ROI Descriptor (Inner Find Circular Edge 2)"=w322, "Fitted Circle (Otter-Find Circular Edge)"=w321) -> ("Roi"=w319:T11, "New Inneer ROI"=w315:T1)  [unwired: 8 in]
      n61 = call "Inner Center13"("Image In"=w318, "ROI Descriptor (Inner Find Circular Edge 2)"=w315, "Options (Inner Find Circular Edge 2)"=w328) -> ("Image Out"=w327:T5, "Fitted Circle (Inner Find Circular Edge 2)"=w320:T10)  [unwired: 21 in, 2 out]
      n62 = call "KB-CalRoi_Inner.vi"("Inner ROI Descriptor (Inner Find Circular Edge 2)"=w315, "Fitted Circle (Otter-Find Circular Edge)"=w320) -> ()  [unwired: 8 in, 2 out]
    }
    frame "Item15" {
      (unwired) cluster{"Lower value":sgl, "Upper value":sgl} {"Lower value"=96.0, "Upper value"=255.0} ("Range (Threshold 1)")
      n63 = call "Out Center15"("Image In"=w341, "ROI Descriptor (Otter-Find Circular Edge)"=w340, "Options (Otter-Find Circular Edge)"=w339, "Range (Threshold 1)"=w331, "Circle Fit Options (Otter-Find Circular Edge)"=T9 {"Process"=enum."Get Best Edge", "Step Size"=10, "Max Pixel Radius"=13}, "error in"=w338) -> ("Fitted Circle (Otter-Find Circular Edge)"=w336:T10)  [unwired: 19 in, 2 out]
      n64 = call "KB-CalRoi_Inner.vi"("Inner ROI Descriptor (Inner Find Circular Edge 2)"=w337, "Fitted Circle (Otter-Find Circular Edge)"=w336) -> ("Roi"=w333:T11, "New Inneer ROI"=w330:T1)  [unwired: 8 in]
      n65 = call "Inner Center14"("Image In"=w334, "ROI Descriptor (Inner Find Circular Edge 2)"=w330, "Options (Inner Find Circular Edge 2)"=w343) -> ("Image Out"=w342:T5, "Fitted Circle (Inner Find Circular Edge 2)"=w335:T10)  [unwired: 21 in, 2 out]
      n66 = call "KB-CalRoi_Inner.vi"("Inner ROI Descriptor (Inner Find Circular Edge 2)"=w330, "Fitted Circle (Otter-Find Circular Edge)"=w335) -> ()  [unwired: 8 in, 2 out]
    }
    frame "Item16" {
      (unwired) cluster{"Lower value":sgl, "Upper value":sgl} {"Lower value"=98.0, "Upper value"=255.0} ("Range (Threshold 1)")
      n67 = call "Out Center16"("Image In"=w357, "ROI Descriptor (Otter-Find Circular Edge)"=w356, "Options (Otter-Find Circular Edge)"=w355, "Range (Threshold 1)"=w347, "Circle Fit Options (Otter-Find Circular Edge)"=T9 {"Process"=enum."Get Best Edge", "Step Size"=10, "Max Pixel Radius"=13}, "error in"=w354) -> ("Image Out"=w346:T5, "Fitted Circle (Otter-Find Circular Edge)"=w352:T10)  [unwired: 19 in, 1 out]
      n68 = call "KB-CalRoi_Inner.vi"("Inner ROI Descriptor (Inner Find Circular Edge 2)"=w353, "Fitted Circle (Otter-Find Circular Edge)"=w352) -> ("Roi"=w349:T11, "New Inneer ROI"=w345:T1)  [unwired: 8 in]
      n69 = call "Inner Center15"("Image In"=w350, "ROI Descriptor (Inner Find Circular Edge 2)"=w345, "Options (Inner Find Circular Edge 2)"=w359) -> ("Image Out"=w358:T5, "Fitted Circle (Inner Find Circular Edge 2)"=w351:T10)  [unwired: 21 in, 2 out]
      n70 = call "KB-CalRoi_Inner.vi"("Inner ROI Descriptor (Inner Find Circular Edge 2)"=w345, "Fitted Circle (Otter-Find Circular Edge)"=w351) -> ()  [unwired: 8 in, 2 out]
    }
    frame "Item17" {
      (unwired) cluster{"Lower value":sgl, "Upper value":sgl} {"Lower value"=156.0, "Upper value"=255.0} ("Range (Threshold 1)")
      n71 = call "Out Center17"("Image In"=w372, "ROI Descriptor (Otter-Find Circular Edge)"=w371, "Options (Otter-Find Circular Edge)"=w370, "Range (Threshold 1)"=w362, "Circle Fit Options (Otter-Find Circular Edge)"=T9 {"Process"=enum."Get Best Edge", "Step Size"=10, "Max Pixel Radius"=13}, "error in"=w369) -> ("Fitted Circle (Otter-Find Circular Edge)"=w367:T10)  [unwired: 19 in, 2 out]
      n72 = call "KB-CalRoi_Inner.vi"("Inner ROI Descriptor (Inner Find Circular Edge 2)"=w368, "Fitted Circle (Otter-Find Circular Edge)"=w367) -> ("Roi"=w365:T11, "New Inneer ROI"=w361:T1)  [unwired: 8 in]
      n73 = call "Inner Center16"("Image In"=w364, "ROI Descriptor (Inner Find Circular Edge 2)"=w361, "Options (Inner Find Circular Edge 2)"=w374) -> ("Image Out"=w373:T5, "Fitted Circle (Inner Find Circular Edge 2)"=w366:T10)  [unwired: 21 in, 2 out]
      n74 = call "KB-CalRoi_Inner.vi"("Inner ROI Descriptor (Inner Find Circular Edge 2)"=w361, "Fitted Circle (Otter-Find Circular Edge)"=w366) -> ()  [unwired: 8 in, 2 out]
    }
    frame "Item18" {
      (unwired) cluster{"Lower value":sgl, "Upper value":sgl} {"Lower value"=197.0, "Upper value"=255.0} ("Range (Threshold 1)")
      n75 = call "Out Center18"("Image In"=w388, "ROI Descriptor (Otter-Find Circular Edge)"=w387, "Options (Otter-Find Circular Edge)"=w386, "Range (Threshold 1)"=w378, "Circle Fit Options (Otter-Find Circular Edge)"=T9 {"Process"=enum."Get Best Edge", "Step Size"=10, "Max Pixel Radius"=13}, "error in"=w385) -> ("Image Out"=w377:T5, "Fitted Circle (Otter-Find Circular Edge)"=w383:T10)  [unwired: 19 in, 1 out]
      n76 = call "KB-CalRoi_Inner.vi"("Inner ROI Descriptor (Inner Find Circular Edge 2)"=w384, "Fitted Circle (Otter-Find Circular Edge)"=w383) -> ("Roi"=w381:T11, "New Inneer ROI"=w376:T1)  [unwired: 8 in]
      n77 = call "Inner Center17"("Image In"=w380, "ROI Descriptor (Inner Find Circular Edge 2)"=w376, "Options (Inner Find Circular Edge 2)"=w390) -> ("Image Out"=w389:T5, "Fitted Circle (Inner Find Circular Edge 2)"=w382:T10)  [unwired: 21 in, 2 out]
      n78 = call "KB-CalRoi_Inner.vi"("Inner ROI Descriptor (Inner Find Circular Edge 2)"=w376, "Fitted Circle (Otter-Find Circular Edge)"=w382) -> ()  [unwired: 8 in, 2 out]
    }
    frame "Item19" {
      (unwired) cluster{"Lower value":sgl, "Upper value":sgl} {"Lower value"=187.0, "Upper value"=255.0} ("Range (Threshold 1)")
      n79 = call "Out Center19"("Image In"=w404, "ROI Descriptor (Otter-Find Circular Edge)"=w403, "Options (Otter-Find Circular Edge)"=w402, "Range (Threshold 1)"=w394, "Circle Fit Options (Otter-Find Circular Edge)"=T9 {"Process"=enum."Get Best Edge", "Step Size"=10, "Max Pixel Radius"=13}, "error in"=w401) -> ("Image Out"=w393:T5, "Fitted Circle (Otter-Find Circular Edge)"=w399:T10)  [unwired: 19 in, 1 out]
      n80 = call "KB-CalRoi_Inner.vi"("Inner ROI Descriptor (Inner Find Circular Edge 2)"=w400, "Fitted Circle (Otter-Find Circular Edge)"=w399) -> ("Roi"=w396:T11, "New Inneer ROI"=w392:T1)  [unwired: 8 in]
      n81 = call "Inner Center18"("Image In"=w397, "ROI Descriptor (Inner Find Circular Edge 2)"=w392, "Options (Inner Find Circular Edge 2)"=w406) -> ("Image Out"=w405:T5, "Fitted Circle (Inner Find Circular Edge 2)"=w398:T10)  [unwired: 21 in, 2 out]
      n82 = call "KB-CalRoi_Inner.vi"("Inner ROI Descriptor (Inner Find Circular Edge 2)"=w392, "Fitted Circle (Otter-Find Circular Edge)"=w398) -> ()  [unwired: 8 in, 2 out]
    }
    frame "Item20" {
      (unwired) cluster{"Lower value":sgl, "Upper value":sgl} {"Lower value"=211.0, "Upper value"=255.0} ("Range (Threshold 1)")
      n83 = call "Out Center20"("Image In"=w420, "ROI Descriptor (Otter-Find Circular Edge)"=w419, "Options (Otter-Find Circular Edge)"=w418, "Range (Threshold 1)"=w410, "Circle Fit Options (Otter-Find Circular Edge)"=T9 {"Process"=enum."Get Best Edge", "Step Size"=10, "Max Pixel Radius"=13}, "error in"=w417) -> ("Image Out"=w409:T5, "Fitted Circle (Otter-Find Circular Edge)"=w415:T10)  [unwired: 19 in, 1 out]
      n84 = call "KB-CalRoi_Inner.vi"("Inner ROI Descriptor (Inner Find Circular Edge 2)"=w416, "Fitted Circle (Otter-Find Circular Edge)"=w415) -> ("Roi"=w412:T11, "New Inneer ROI"=w408:T1)  [unwired: 8 in]
      n85 = call "Inner Center19"("Image In"=w413, "ROI Descriptor (Inner Find Circular Edge 2)"=w408, "Options (Inner Find Circular Edge 2)"=w422) -> ("Image Out"=w421:T5, "Fitted Circle (Inner Find Circular Edge 2)"=w414:T10)  [unwired: 21 in, 2 out]
      n86 = call "KB-CalRoi_Inner.vi"("Inner ROI Descriptor (Inner Find Circular Edge 2)"=w408, "Fitted Circle (Otter-Find Circular Edge)"=w414) -> ()  [unwired: 8 in, 2 out]
    }
    frame "Item21" {
      (unwired) cluster{"Lower value":sgl, "Upper value":sgl} {"Lower value"=188.0, "Upper value"=255.0} ("Range (Threshold 1)")
      n87 = call "Out Center21"("Image In"=w436, "ROI Descriptor (Otter-Find Circular Edge)"=w435, "Options (Otter-Find Circular Edge)"=w434, "Range (Threshold 1)"=w426, "Circle Fit Options (Otter-Find Circular Edge)"=T9 {"Process"=enum."Get Best Edge", "Step Size"=10, "Max Pixel Radius"=13}, "error in"=w433) -> ("Image Out"=w425:T5, "Fitted Circle (Otter-Find Circular Edge)"=w431:T10)  [unwired: 19 in, 1 out]
      n88 = call "KB-CalRoi_Inner.vi"("Inner ROI Descriptor (Inner Find Circular Edge 2)"=w432, "Fitted Circle (Otter-Find Circular Edge)"=w431) -> ("Roi"=w428:T11, "New Inneer ROI"=w424:T1)  [unwired: 8 in]
      n89 = call "Inner Center20"("Image In"=w429, "ROI Descriptor (Inner Find Circular Edge 2)"=w424, "Options (Inner Find Circular Edge 2)"=w438) -> ("Image Out"=w437:T5, "Fitted Circle (Inner Find Circular Edge 2)"=w430:T10)  [unwired: 21 in, 2 out]
      n90 = call "KB-CalRoi_Inner.vi"("Inner ROI Descriptor (Inner Find Circular Edge 2)"=w424, "Fitted Circle (Otter-Find Circular Edge)"=w430) -> ()  [unwired: 8 in, 2 out]
    }
    frame "Item22" {
      n91 = call "Out Center"("Image In"=w455, "ROI Descriptor (Otter-Find Circular Edge)"=w454, "Options (Otter-Find Circular Edge)"=w453, "Circle Fit Options (Otter-Find Circular Edge)"=T9 {"Process"=enum."Get Best Edge", "Step Size"=10, "Max Pixel Radius"=13}, "Red or Hue Range (Color Threshold 1)"=w444, "Green or Sat Range (Color Threshold 1)"=w444, "error in"=w452, "Blue or Luma or Val or Inten Range (Color Threshold 1)"=w444) -> ("Fitted Circle (Otter-Find Circular Edge)"=w450:T10, "error out"=w446:errorcluster)  [unwired: 17 in, 1 out]
      n92 = call "KB-CalRoi_Inner.vi"("Inner ROI Descriptor (Inner Find Circular Edge 2)"=w451, "Fitted Circle (Otter-Find Circular Edge)"=w450) -> ("Roi"=w442:T11, "New Inneer ROI"=w443:T1)  [unwired: 8 in]
      n93 = call "Inner Center22"("Image In"=w448, "Circle Fit Options (Inner Find Circular Edge 2)"=T9 {"Process"=enum."Get Best Edge", "Step Size"=10, "Max Pixel Radius"=3}, "ROI Descriptor (Inner Find Circular Edge 2)"=w443, "Options (Inner Find Circular Edge 2)"=w456, "error in"=w446) -> ("Image Out"=w441:T5, "Fitted Circle (Inner Find Circular Edge 2)"=w449:T10, "error out"=w440:errorcluster)  [unwired: 19 in, 1 out]
      n94 = call "KB-CalRoi_Inner.vi"("Inner ROI Descriptor (Inner Find Circular Edge 2)"=w443, "Fitted Circle (Otter-Find Circular Edge)"=w449) -> ()  [unwired: 8 in, 2 out]
    }
    frame "Item23" {
      n95 = call "Out Center23"("Image In"=w463, "ROI Descriptor (Otter-Find Circular Edge)"=w473, "Options (Otter-Find Circular Edge)"=w472, "Circle Fit Options (Otter-Find Circular Edge)"=T9 {"Process"=enum."Get First + Last Edge", "Step Size"=10, "Max Pixel Radius"=13}, "Range (Threshold 1)"=w464, "error in"=w471) -> ("Fitted Circle (Otter-Find Circular Edge)"=w469:T10, "error out"=w468:errorcluster)  [unwired: 19 in, 1 out]
      n96 = call "KB-CalRoi_Inner.vi"("Inner ROI Descriptor (Inner Find Circular Edge 2)"=w470, "Fitted Circle (Otter-Find Circular Edge)"=w469) -> ("Roi"=w458:T11, "New Inneer ROI"=w461:T1)  [unwired: 8 in]
      n97 = call "Inner Center23"("Image In"=w465, "Circle Fit Options (Inner Find Circular Edge 2)"=T9 {"Process"=enum."Get Best Edge", "Step Size"=10, "Max Pixel Radius"=13}, "ROI Descriptor (Inner Find Circular Edge 2)"=w461, "Options (Inner Find Circular Edge 2)"=w474, "error in"=w468) -> ("Image Out"=w459:T5, "Fitted Circle (Inner Find Circular Edge 2)"=w462:T10, "error out"=w460:errorcluster)  [unwired: 19 in, 1 out]
      n98 = call "KB-CalRoi_Inner.vi"("Inner ROI Descriptor (Inner Find Circular Edge 2)"=w461, "Fitted Circle (Otter-Find Circular Edge)"=w462) -> ()  [unwired: 8 in, 2 out]
    }
    frame "Item24" {
      n99 = call "Out Center24"("Image In"=w491, "ROI Descriptor (Otter-Find Circular Edge)"=w490, "Options (Otter-Find Circular Edge)"=w489, "Circle Fit Options (Otter-Find Circular Edge)"=T9 {"Process"=enum."Get First + Last Edge", "Step Size"=10, "Max Pixel Radius"=13}, "Red or Hue Range (Color Threshold 1)"=w480, "Green or Sat Range (Color Threshold 1)"=w480, "error in"=w488, "Blue or Luma or Val or Inten Range (Color Threshold 1)"=w480) -> ("Fitted Circle (Otter-Find Circular Edge)"=w486:T10, "error out"=w483:errorcluster)  [unwired: 17 in, 1 out]
      n100 = call "KB-CalRoi_Inner.vi"("Inner ROI Descriptor (Inner Find Circular Edge 2)"=w487, "Fitted Circle (Otter-Find Circular Edge)"=w486) -> ("Roi"=w478:T11, "New Inneer ROI"=w479:T1)  [unwired: 8 in]
      n101 = call "Inner Center24"("Image In"=w484, "Circle Fit Options (Inner Find Circular Edge 2)"=T9 {"Process"=enum."Get Best Edge", "Step Size"=10, "Max Pixel Radius"=13}, "ROI Descriptor (Inner Find Circular Edge 2)"=w479, "Options (Inner Find Circular Edge 2)"=w492, "error in"=w483) -> ("Image Out"=w477:T5, "Fitted Circle (Inner Find Circular Edge 2)"=w485:T10, "error out"=w476:errorcluster)  [unwired: 19 in, 1 out]
      n102 = call "KB-CalRoi_Inner.vi"("Inner ROI Descriptor (Inner Find Circular Edge 2)"=w479, "Fitted Circle (Otter-Find Circular Edge)"=w485) -> ()  [unwired: 8 in, 2 out]
    }
    frame "Item25" {
      n103 = call "Out Center25"("Image In"=w509, "ROI Descriptor (Otter-Find Circular Edge)"=w508, "Options (Otter-Find Circular Edge)"=w507, "Circle Fit Options (Otter-Find Circular Edge)"=T9 {"Process"=enum."Get First + Last Edge", "Step Size"=10, "Max Pixel Radius"=13}, "Red or Hue Range (Color Threshold 1)"=w498, "Green or Sat Range (Color Threshold 1)"=w498, "error in"=w506, "Blue or Luma or Val or Inten Range (Color Threshold 1)"=w498) -> ("Fitted Circle (Otter-Find Circular Edge)"=w504:T10, "error out"=w502:errorcluster)  [unwired: 17 in, 1 out]
      n104 = call "KB-CalRoi_Inner.vi"("Inner ROI Descriptor (Inner Find Circular Edge 2)"=w505, "Fitted Circle (Otter-Find Circular Edge)"=w504) -> ("Roi"=w494:T11, "New Inneer ROI"=w497:T1)  [unwired: 8 in]
      n105 = call "Inner Center25"("Image In"=w501, "Circle Fit Options (Inner Find Circular Edge 2)"=T9 {"Process"=enum."Get Best Edge", "Step Size"=10, "Max Pixel Radius"=13}, "ROI Descriptor (Inner Find Circular Edge 2)"=w497, "Options (Inner Find Circular Edge 2)"=w510, "error in"=w502) -> ("Image Out"=w495:T5, "Fitted Circle (Inner Find Circular Edge 2)"=w503:T10, "error out"=w496:errorcluster)  [unwired: 19 in, 1 out]
      n106 = call "KB-CalRoi_Inner.vi"("Inner ROI Descriptor (Inner Find Circular Edge 2)"=w497, "Fitted Circle (Otter-Find Circular Edge)"=w503) -> ()  [unwired: 8 in, 2 out]
    }
    frame "Item26" {
      n107 = call "Out Center26"("Image In"=w527, "ROI Descriptor (Otter-Find Circular Edge)"=w526, "Options (Otter-Find Circular Edge)"=w525, "Circle Fit Options (Otter-Find Circular Edge)"=T9 {"Process"=enum."Get First + Last Edge", "Step Size"=10, "Max Pixel Radius"=13}, "Red or Hue Range (Color Threshold 1)"=w516, "Green or Sat Range (Color Threshold 1)"=w516, "error in"=w524, "Blue or Luma or Val or Inten Range (Color Threshold 1)"=w516) -> ("Fitted Circle (Otter-Find Circular Edge)"=w522:T10, "error out"=w523:errorcluster)  [unwired: 17 in, 1 out]
      n108 = call "KB-CalRoi_Inner.vi"("Inner ROI Descriptor (Inner Find Circular Edge 2)"=w515, "Fitted Circle (Otter-Find Circular Edge)"=w522) -> ("Roi"=w514:T11, "New Inneer ROI"=w521:T1)  [unwired: 8 in]
      n109 = call "Inner Center26"("Image In"=w518, "Circle Fit Options (Inner Find Circular Edge 2)"=T9 {"Process"=enum."Get Best Edge", "Step Size"=10, "Max Pixel Radius"=3}, "ROI Descriptor (Inner Find Circular Edge 2)"=w521, "Options (Inner Find Circular Edge 2)"=w528, "error in"=w523) -> ("Image Out"=w513:T5, "Fitted Circle (Inner Find Circular Edge 2)"=w520:T10, "error out"=w512:errorcluster)  [unwired: 19 in, 1 out]
      n110 = call "KB-CalRoi_Inner.vi"("Inner ROI Descriptor (Inner Find Circular Edge 2)"=w515, "Fitted Circle (Otter-Find Circular Edge)"=w520) -> ()  [unwired: 8 in, 2 out]
    }
    frame "Item27" {
      n111 = call "Out Center27"("Image In"=w544, "ROI Descriptor (Otter-Find Circular Edge)"=w543, "Options (Otter-Find Circular Edge)"=w542, "Circle Fit Options (Otter-Find Circular Edge)"=T9 {"Process"=enum."Get First + Last Edge", "Step Size"=10, "Max Pixel Radius"=13}, "Red or Hue Range (Color Threshold 1)"=w534, "Green or Sat Range (Color Threshold 1)"=w534, "error in"=w541, "Blue or Luma or Val or Inten Range (Color Threshold 1)"=w534) -> ("Fitted Circle (Otter-Find Circular Edge)"=w539:T10)  [unwired: 17 in, 2 out]
      n112 = call "KB-CalRoi_Inner.vi"("Inner ROI Descriptor (Inner Find Circular Edge 2)"=w540, "Fitted Circle (Otter-Find Circular Edge)"=w539) -> ("Roi"=w532:T11, "New Inneer ROI"=w533:T1)  [unwired: 8 in]
      n113 = call "Inner Center27"("Image In"=w537, "Circle Fit Options (Inner Find Circular Edge 2)"=T9 {"Process"=enum."Get Best Edge", "Step Size"=10, "Max Pixel Radius"=3}, "ROI Descriptor (Inner Find Circular Edge 2)"=w533, "Options (Inner Find Circular Edge 2)"=w545) -> ("Image Out"=w530:T5, "Fitted Circle (Inner Find Circular Edge 2)"=w538:T10, "error out"=w531:errorcluster)  [unwired: 20 in, 1 out]
      n114 = call "KB-CalRoi_Inner.vi"("Inner ROI Descriptor (Inner Find Circular Edge 2)"=w533, "Fitted Circle (Otter-Find Circular Edge)"=w538) -> ()  [unwired: 8 in, 2 out]
    }
    frame "Item28" {
      n115 = call "Out Center28"("Image In"=w561, "ROI Descriptor (Otter-Find Circular Edge)"=w560, "Options (Otter-Find Circular Edge)"=w559, "Circle Fit Options (Otter-Find Circular Edge)"=T9 {"Process"=enum."Get First + Last Edge", "Step Size"=10, "Max Pixel Radius"=13}, "Red or Hue Range (Color Threshold 1)"=w551, "Green or Sat Range (Color Threshold 1)"=w551, "error in"=w558, "Blue or Luma or Val or Inten Range (Color Threshold 1)"=w551) -> ("Fitted Circle (Otter-Find Circular Edge)"=w556:T10)  [unwired: 17 in, 2 out]
      n116 = call "KB-CalRoi_Inner.vi"("Inner ROI Descriptor (Inner Find Circular Edge 2)"=w557, "Fitted Circle (Otter-Find Circular Edge)"=w556) -> ("Roi"=w549:T11, "New Inneer ROI"=w550:T1)  [unwired: 8 in]
      n117 = call "Inner Center28"("Image In"=w554, "Circle Fit Options (Inner Find Circular Edge 2)"=T9 {"Process"=enum."Get Best Edge", "Step Size"=10, "Max Pixel Radius"=3}, "ROI Descriptor (Inner Find Circular Edge 2)"=w550, "Options (Inner Find Circular Edge 2)"=w562) -> ("Image Out"=w547:T5, "Fitted Circle (Inner Find Circular Edge 2)"=w555:T10, "error out"=w548:errorcluster)  [unwired: 20 in, 1 out]
      n118 = call "KB-CalRoi_Inner.vi"("Inner ROI Descriptor (Inner Find Circular Edge 2)"=w550, "Fitted Circle (Otter-Find Circular Edge)"=w555) -> ()  [unwired: 8 in, 2 out]
    }
    frame "Item29" {
      n119 = call "Out Center29"("Image In"=w578, "ROI Descriptor (Otter-Find Circular Edge)"=w577, "Options (Otter-Find Circular Edge)"=w576, "Circle Fit Options (Otter-Find Circular Edge)"=T9 {"Process"=enum."Get First + Last Edge", "Step Size"=10, "Max Pixel Radius"=13}, "Red or Hue Range (Color Threshold 1)"=w568, "Green or Sat Range (Color Threshold 1)"=w568, "error in"=w575, "Blue or Luma or Val or Inten Range (Color Threshold 1)"=w568) -> ("Fitted Circle (Otter-Find Circular Edge)"=w573:T10)  [unwired: 17 in, 2 out]
      n120 = call "KB-CalRoi_Inner.vi"("Inner ROI Descriptor (Inner Find Circular Edge 2)"=w574, "Fitted Circle (Otter-Find Circular Edge)"=w573) -> ("Roi"=w566:T11, "New Inneer ROI"=w567:T1)  [unwired: 8 in]
      n121 = call "Inner Center29"("Image In"=w570, "Circle Fit Options (Inner Find Circular Edge 2)"=T9 {"Process"=enum."Get Best Edge", "Step Size"=10, "Max Pixel Radius"=3}, "ROI Descriptor (Inner Find Circular Edge 2)"=w567, "Options (Inner Find Circular Edge 2)"=w579) -> ("Image Out"=w565:T5, "error out"=w564:errorcluster, "Fitted Circle (Inner Find Circular Edge 2)"=w572:T10)  [unwired: 20 in, 1 out]
      n122 = call "KB-CalRoi_Inner.vi"("Inner ROI Descriptor (Inner Find Circular Edge 2)"=w567, "Fitted Circle (Otter-Find Circular Edge)"=w572) -> ()  [unwired: 8 in, 2 out]
    }
    frame "Item30" {
      n123 = call "Out Center30"("Image In"=w595, "ROI Descriptor (Otter-Find Circular Edge)"=w594, "Options (Otter-Find Circular Edge)"=w593, "Circle Fit Options (Otter-Find Circular Edge)"=T9 {"Process"=enum."Get First + Last Edge", "Step Size"=10, "Max Pixel Radius"=13}, "Red or Hue Range (Color Threshold 1)"=w585, "Green or Sat Range (Color Threshold 1)"=w585, "error in"=w592, "Blue or Luma or Val or Inten Range (Color Threshold 1)"=w585) -> ("Fitted Circle (Otter-Find Circular Edge)"=w590:T10)  [unwired: 17 in, 2 out]
      n124 = call "KB-CalRoi_Inner.vi"("Inner ROI Descriptor (Inner Find Circular Edge 2)"=w591, "Fitted Circle (Otter-Find Circular Edge)"=w590) -> ("Roi"=w581:T11, "New Inneer ROI"=w584:T1)  [unwired: 8 in]
      n125 = call "Inner Center30"("Image In"=w587, "Circle Fit Options (Inner Find Circular Edge 2)"=T9 {"Process"=enum."Get Best Edge", "Step Size"=10, "Max Pixel Radius"=3}, "ROI Descriptor (Inner Find Circular Edge 2)"=w584, "Options (Inner Find Circular Edge 2)"=w596) -> ("Image Out"=w583:T5, "error out"=w582:errorcluster, "Fitted Circle (Inner Find Circular Edge 2)"=w589:T10)  [unwired: 20 in, 1 out]
      n126 = call "KB-CalRoi_Inner.vi"("Inner ROI Descriptor (Inner Find Circular Edge 2)"=w584, "Fitted Circle (Otter-Find Circular Edge)"=w589) -> ()  [unwired: 8 in, 2 out]
    }
    frame "Item31" {
      n127 = call "Out Center31"("Image In"=w613, "ROI Descriptor (Otter-Find Circular Edge)"=w612, "Options (Otter-Find Circular Edge)"=w611, "Circle Fit Options (Otter-Find Circular Edge)"=T9 {"Process"=enum."Get Best Edge", "Step Size"=10, "Max Pixel Radius"=13}, "Range (Threshold 1)"=w602, "error in"=w610) -> ("Fitted Circle (Otter-Find Circular Edge)"=w608:T10, "error out"=w605:errorcluster)  [unwired: 19 in, 1 out]
      n128 = call "KB-CalRoi_Inner.vi"("Inner ROI Descriptor (Inner Find Circular Edge 2)"=w609, "Fitted Circle (Otter-Find Circular Edge)"=w608) -> ("Roi"=w600:T11, "New Inneer ROI"=w601:T1)  [unwired: 8 in]
      n129 = call "Inner Center31"("Image In"=w603, "Circle Fit Options (Inner Find Circular Edge 2)"=T9 {"Process"=enum."Get Best Edge", "Step Size"=10, "Max Pixel Radius"=3}, "ROI Descriptor (Inner Find Circular Edge 2)"=w601, "Options (Inner Find Circular Edge 2)"=w614, "error in"=w605) -> ("Image Out"=w598:T5, "Fitted Circle (Inner Find Circular Edge 2)"=w607:T10, "error out"=w599:errorcluster)  [unwired: 19 in, 1 out]
      n130 = call "KB-CalRoi_Inner.vi"("Inner ROI Descriptor (Inner Find Circular Edge 2)"=w601, "Fitted Circle (Otter-Find Circular Edge)"=w607) -> ()  [unwired: 8 in, 2 out]
    }
  }
  "New Inneer ROI 2" <- w7
  n131 = Build Array (concatenate)(w59, 0) -> (w57:i32[])
  n132 = Bundle By Name(cluster=T8 {"ID"=enum."External", "Type"=12, "Coordinates"=[726, 409, 3048, 1749, 0]}, "Coordinates"=w57) -> (w56:T8)
  n133 = Build Array(w56) -> (w55:T12)
  n134 = Bundle By Name(cluster=T1 {"Global Rectangle"=[726, 409, 3048, 1749], "Contours"=[{"ID"=enum."External", "Type"=12, "Coordinates"=[726, 409, 3048, 1749, 0]}]} ("ROI Descriptor (Color Pattern Matching 1)"), "Global Rectangle"=w59, "Contours"=w55) -> (→"New Inneer ROI":T1)
  n135 = Unbundle By Name(w76) -> ("Center (Pixels)"=w66:cluster{"X":sgl, "Y":sgl}, "Center (Pixels).X"=w75:sgl, "Center (Pixels).Y"=w74:sgl)
  n136 = global read "Global System.vi" "ref path"() -> (w41:path)
  n137 = Unbundle By Name(w7) -> ("Global Rectangle"=w32:i32[])
  n138 = call "IMAQ Overlay Oval"("Color"=u32 16711680, "Drawing Mode (Frame)"=w40, "Bounding Rectangle"=w38, "Image"=w5) -> ("error out"=w15:errorcluster, "Image Out"=w18:T5)  [unwired: 6 in]
  n139 = Unbundle By Name(w73) -> ("Center (Pixels)"=w65:cluster{"X":sgl, "Y":sgl}, "Center (Pixels).X"=w72:sgl, "Center (Pixels).Y"=w71:sgl)
  n140 = call <vilib>:"Clear Errors.vi"("error in (no error)"=w14) -> ("error out"=w10:errorcluster)  [unwired: 5 in, 1 out]
  n141 = call "时间延迟"("error in (no error)"=w10, "Delay Time (s)"=0.0) -> ("error out"=w11:errorcluster)  [unwired: 9 in]
  n142 = call "IPI_DrawCross.vi"("Image In"=w18, "X"=w75, "Y"=w74, "error in (no error)"=w15, "Radius"=w70, "颜色盒"=w69) -> ("Image Out"=w49:T5, "error out"=w68:errorcluster)  [unwired: 8 in]
  n143 = Build Path(base path=w41, name or relative path=w19) -> (appended path=w8:path)
  n144 = Fract/Exp String To Number(string="相机分辨率", default (0 dbl)=10.0 ("默认(0 DBL)")) -> (number=w84:dbl)  [unwired: 2 in, 1 out]
  n145 = call "KB-Cal-Distance.vi"("Fitted Circle (Inner Find Circular Edge 2)"=w73, "Fitted Circle (Otter-Find Circular Edge)"=w76) -> ("Distance"=w77:sgl)  [unwired: 9 in]
  n146 = call "color 1.vi"("ROI Descriptor"=w7, "Image 2"=w5, "color"=w8) -> ("Class"=→"color":string)  [unwired: 7 in, 1 out]
  n147 = Multiply(x=w77, y=w84) -> (x*y=w35:dbl)
  n148 = Index Array(array=w32) -> (element #1=w29:i32, element #2=w28:i32, element #3=w27:i32, element #4=w26:i32)  [unwired: 4 in]
  n149 = Greater Or Equal?(x=w35, y=0.2) -> (x >= y?=w36:bool)
  n150 = call "IPI_DrawCross.vi"("Image In"=w49, "X"=w72, "Y"=w71, "error in (no error)"=w68, "Radius"=w70, "颜色盒"=w69) -> ("Image Out"=w67:T5, "error out"=w64:errorcluster)  [unwired: 8 in]
  n151 = disable-structure shown="禁用" {
    disable-tunnel: [w619 _] -> w43
    disable-tunnel: w11 -> [w618 _]
    disable-tunnel: w8 -> [w617 _]
    disable-tunnel: w7 -> [w616 _]
    frame Disabled {
      n152 = call "Vision Assistant"("File Path (Color Classification 1)"=w617, "ROI Descriptor (Color Classification 1)"=w616, "error in"=w618) -> ("Classes (Color Classification 1)"=w619:string[])  [unwired: 22 in, 2 out]
    }
    frame Enabled {
    }
  }
  n153 = case shown="真" w36 {
    tunnel: w35 -> [w620 w625]
    tunnel: [w620 w621] -> w34
    frame False {
    }
    frame True {
      n154 = Random Number (0-1)() -> (number: 0 to 1=w623:dbl)
      n155 = Divide(x=w625, y=3.0) -> ()  [unwired: 1 out]
      n156 = Divide(x=w623, y=10.0) -> (x/y=w621:dbl)
    }
  }
  n157 = Multiply(x=w34, y=1.0) -> (x*y=w52:dbl)
  n158 = Divide(x=w52, y=1.0) -> (x/y=w50:dbl)
  n159 = case shown="\"假\", 默认" "Row Select" {
    tunnel: [w628 "0" "0" "0" "0"] -> w2
    tunnel: w50 -> [w626 _ _ _ _]
    frame "假", Default {
      n160 = Number To Fractional String(number=w626, precision (6)=i16 3 ("精度(6)")) -> (F-format string=w629:string)  [unwired: 2 in]
      n161 = Concatenate Strings(w629) -> (w628:string)
    }
    frame "Item7" {
    }
    frame "Item9" {
    }
    frame "Item10" {
    }
    frame "Item8" {
    }
  }
  n162 = Bundle By Name(cluster=T6 {"Left"=0, "Top"=0, "Right"=0, "Bottom"=0} ("Rectangle"), "Left"=w29, "Top"=w28, "Right"=w27, "Bottom"=w26) -> (w25:T6)
  n163 = call "IMAQ Overlay Line"("Color"=u32 6618880, "error in (no error)"=w64, "End Point"=w65, "Start Point"=w66, "Image"=w67) -> ("error out"=w20:errorcluster, "Image Out"=w21:T5)  [unwired: 5 in]
  n164 = call "IMAQ Overlay Rectangle"("Color"=u32 16711680, "error in (no error)"=w20, "Drawing Mode (Frame)"=w24, "Rectangle"=w25, "Image"=w21) -> ("error out"=w22:errorcluster, "Image Out"=→"Image  Out":T5)  [unwired: 5 in]
  n165 = call <vilib>:"Clear Errors.vi"("error in (no error)"=w22) -> ("error out"=→"error out":errorcluster)  [unwired: 5 in, 1 out]
  n166 = Index Array(array=w43, index=0 ("索引")) -> ()  [unwired: 1 out]
  n167 = Unbundle By Name(w76) -> ("Center (Pixels)"=w83:cluster{"X":sgl, "Y":sgl})
  n168 = Unbundle By Name(w73) -> ("Center (Pixels)"=w82:cluster{"X":sgl, "Y":sgl})
  n169 = Equal?(x=w2, y="NaN") -> (x = y?=w3:bool)
  n170 = Build Array(w83, w82) -> (→"U I Center":cluster{"X":sgl, "Y":sgl}[])
  n171 = case shown="假" w3 {
    tunnel: w2 -> [w634 _]
    tunnel: [w634 w635] -> w1
    frame False {
    }
    frame True {
      n172 = Random Number (0-1) "随机数(0-1)"() -> (number: 0 to 1=w641:dbl)
      n173 = Multiply(x=w641, y=2) -> (x*y=w639:dbl)
      n174 = Divide(x=w639, y=10.0) -> (x/y=w636:dbl)
      n175 = Number To Fractional String(number=w636, precision (6)=i16 3 ("精度(6)")) -> (F-format string=w635:string)  [unwired: 2 in]
    }
  }
  "Concentrieity" <- w1
